vi "ALTS-2015 Check & Create Directory.vi"(8 "error in (no error)":errorcluster, 10 "Path is Directory? (F=No)":bool, 11 "Path":path) -> (0 "error out":errorcluster, 3 "Dup Path out":path)   [LabVIEW 2013]
doc: "This VI Check if thegiven directory(s) is available. if the directory is not available, then it creates those directories. If a file path is given it strips the filname and creates the directory.\n\n- Sasikala"
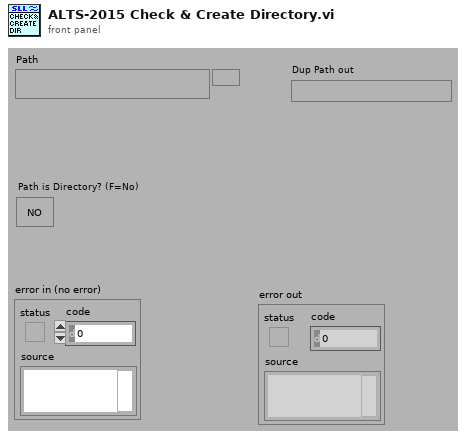
[diagram p1: front panel]
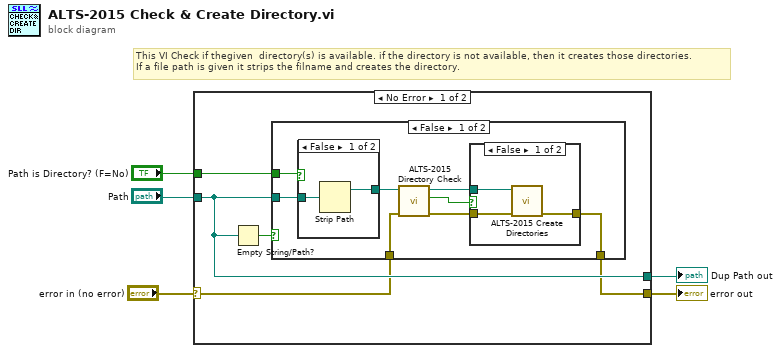
[diagram p0: block diagram]
diagram:
  # "This VI Check if thegiven  directory(s) is available. if the directory is not available, then it creates those directories.\nIf a file path is given it strips the filname and creates the directory."
  n1 = case shown="No Error" "error in (no error)" {
    selector: "error in (no error)" -> [w7 w27]
    tunnel: "Path is Directory? (F=No)" -> [w10 _]
    tunnel: "Path" -> [w8 w28]
    tunnel: [w8 w28] -> w3
    tunnel: [w6 w27] -> w2
    frame No Error {
      n2 = Empty String/Path?(string/path=w8) -> (empty?=w9:bool)
      n3 = case shown="False" w9 {
        tunnel: w10 -> [w18 _]
        tunnel: w8 -> [w17 _]
        tunnel: w7 -> [w13 w26]
        tunnel: [w11 w26] -> w6
        frame False {
          n4 = case shown="False" w18 {
            tunnel: w17 -> [w24 w25]
            tunnel: [w23 w25] -> w14
            frame False {
              n5 = Strip Path(path=w24) -> (stripped path=w23:path)  [unwired: 1 out]
            }
            frame True {
            }
          }
          n6 = call "ALTS-2015 Directory Check.vi"("error in (no error)"=w13, "directory path"=w14) -> ("error out"=w12:errorcluster, "exists?"=w15:bool, "dup directory path"=w16:path)  [unwired: 7 in]
          n7 = case shown="False" w15 {
            tunnel: w16 -> [w21 _]
            tunnel: w12 -> [w20 w22]
            tunnel: [w19 w22] -> w11
            frame False {
              n8 = call "ALTS-2015 Create Directories.vi"("error in (no error)"=w20, "Filepath In"=w21) -> ("error out"=w19:errorcluster)  [unwired: 7 in, 2 out]
            }
            frame True {
            }
          }
        }
        frame True {
        }
      }
    }
    frame Error {
    }
  }
  "Dup Path out" <- w3
  "error out" <- w2
